vi "Transform2d_Create_PosePose.vi"(9 "last POSE":T1 {"ROTATION"."SIN" format="%13.4f"; "ROTATION"."COS" format="%13.4f"; "ROTATION"."VALUE" format="%13.4f"; "TRANSLATION"."Y" format="%14.3f"; "TRANSLATION"."X" format="%14.3f"}, 11 "initial POSE":T1 {"ROTATION"."SIN" format="%13.4f"; "ROTATION"."COS" format="%13.4f"; "ROTATION"."VALUE" format="%13.4f"; "TRANSLATION"."Y" format="%14.3f"; "TRANSLATION"."X" format="%14.3f"}) -> (3 "TRANSFORM":T4 {"ROTATION"."SIN" format="%13.4f"; "ROTATION"."COS" format="%13.4f"; "ROTATION"."VALUE" format="%13.4f"; "TRANSLATION"."Y" format="%14.3f"; "TRANSLATION"."X" format="%14.3f"})   [LabVIEW 2019, in "Trajectory_Library.lvlib"]
doc: "Constructs the transform that maps the initial pose to the final pose.\n\nThis routine rotates the difference between the translations using a clockwise rotation matrix. This transforms the global delta into a local delta (relative to the initial pose).\n\nParameters:\n - initial - The initial pose for the transformation.\n - last - The final pose for the transformation.\n\nReturns:\n - Transform - The TRANSFORM data structure"
uses:
  Trajectory_Library.lvlib
  TRANSLATION2D.ctl
  ROTATION2D.ctl
  TRANSFORM2D.ctl
  POSE2D.ctl
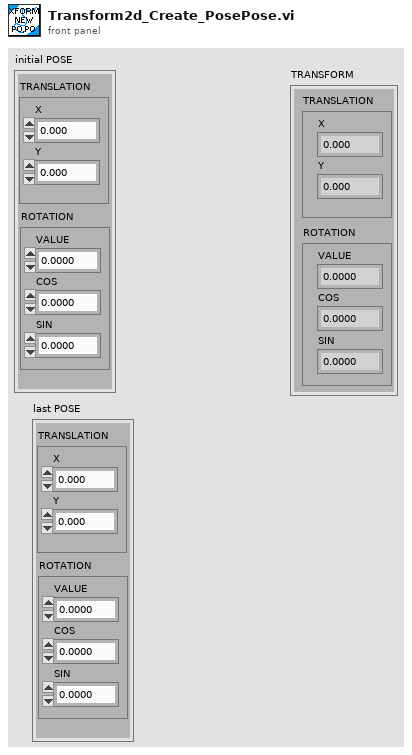
[diagram p1: front panel]
types:
  T1 = typedef "Trajectory_Library.lvlib/POSE2D.ctl" = cluster{"TRANSLATION":T2, "ROTATION":T3}
  T2 = typedef "Trajectory_Library.lvlib/TRANSLATION2D.ctl" = cluster{"X":dbl, "Y":dbl}
  T3 = typedef "Trajectory_Library.lvlib/ROTATION2D.ctl" = cluster{"VALUE":dbl, "COS":dbl, "SIN":dbl}
  T4 = typedef "Trajectory_Library.lvlib/TRANSFORM2D.ctl" = cluster{"TRANSLATION":T2, "ROTATION":T3}
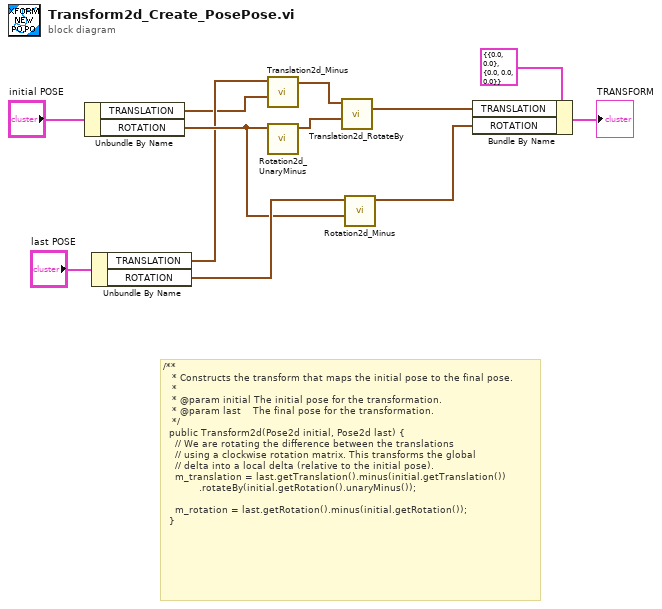
[diagram p0: block diagram]
diagram:
  # "/**\n   * Constructs the transform that maps the initial pose to the final pose.\n   *\n   * @param initial The initial pose for the transformation.\n   * @param last    The final pose for the transformation.\n   */\n  public Transform2d(Pose2d initial, Pose2d last) {\n    // We are rotating the difference between the translations\n    // using a clockwise rotation matrix. This transforms the global\n    // delta into a local delta (relative to the initial pose).\n    m_translation = last.getTranslation().minus(initial.getTranslation())\n            .rotateBy(initial.getRotation().unaryMinus());\n\n    m_rotation = last.getRotation().minus(initial.getRotation());\n  }"
  n1 = Unbundle By Name("initial POSE") -> ("TRANSLATION"=w3:T2, "ROTATION"=w6:T3)
  n2 = Unbundle By Name("last POSE") -> ("TRANSLATION"=w4:T2, "ROTATION"=w7:T3)
  n3 = call "Translation2d_Minus.vi"("other Translation"=w3, "In Translation"=w4) -> ("Out Translation"=w2:T2)  [unwired: 9 in]
  n4 = call "Rotation2d_UnaryMinus.vi"("in ROTATION"=w6) -> ("out ROTATION"=w9:T3)  [unwired: 10 in]
  n5 = call "Translation2d_RotateBy.vi"("other Rotation"=w9, "In Translation"=w2) -> ("Out Translation"=w1:T2)  [unwired: 9 in]
  n6 = call "Rotation2d_Minus.vi"("other ROTATION"=w6, "in ROTATION"=w7) -> ("out ROTATION"=w5:T3)  [unwired: 9 in]
  n7 = Bundle By Name(cluster=T4 {"TRANSLATION"={"X"=0.0, "Y"=0.0}, "ROTATION"={"VALUE"=0.0, "COS"=0.0, "SIN"=0.0}} ("TRANSFORM"), "TRANSLATION"=w1, "ROTATION"=w5) -> (→"TRANSFORM":T4)
